vi "BESSY Put Test.vi"() -> ()   [LabVIEW 2011]
doc: "This Arbitrary Waveform Generator front panel is aimed primarily at the use of two reflectometer instruments at the ISIS Pulsed Neutron Facility at the Rutherford Appleton Laboratory. As such some variable items have been defaulted, and the code follows the standards of the Instrument Controls programming team."
uses:
  Labview Modules/Common/Utilities/Logo.llb/Logo.ctl
  Labview Modules/Common/Utilities/VI Control.llb/Control - Display State.ctl
  Labview Modules/Drivers/Tektronix AFG 3021B/AFG3021B - Controls.llb/AFG3021B - Trigger Button.ctl
  <userlib>/caLab/sub/caLabGet01.vi
  Labview Modules/Common/Utilities/Equal.llb/Equal - Error.vi
  <userlib>/caLab/sub/caLabPut21.vi
panel:
  out "Set Point Ind":dbl
  in  "Set Point":dbl
  in  "Exit":bool
  in  "Set":bool
  out "Message":string
  out "Activity":bool
  out "Error":errorcluster
  in  "Logo":T1
  # "Version 0.0.1"
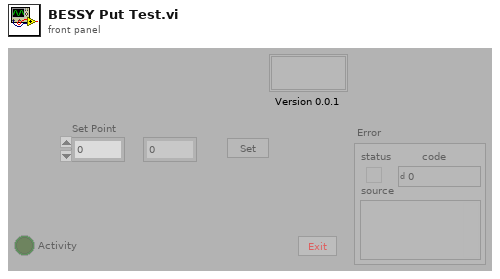
[diagram p1: front panel]
types:
  T1 = typedef "Logo.ctl" = u16
  T2 = typedef "Control - Display State.ctl" = enum16{"Enabled", "Disabled", "Disabled and Grayed"}
  T3 = typedef "AFG3021B - Trigger Button.ctl" = bool
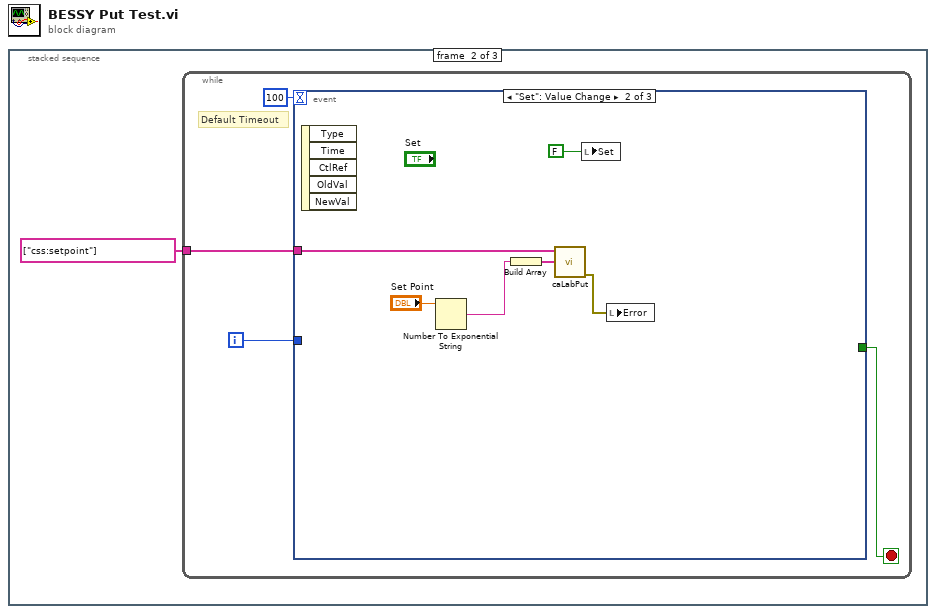
[diagram p0: block diagram]
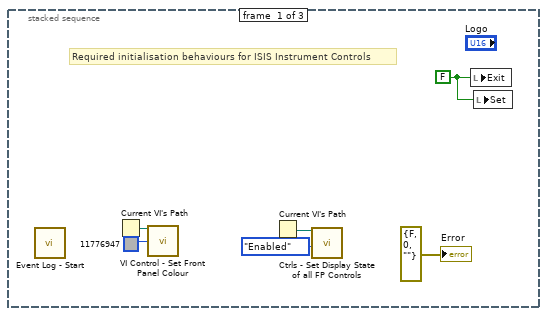
[diagram p2: hidden frame]
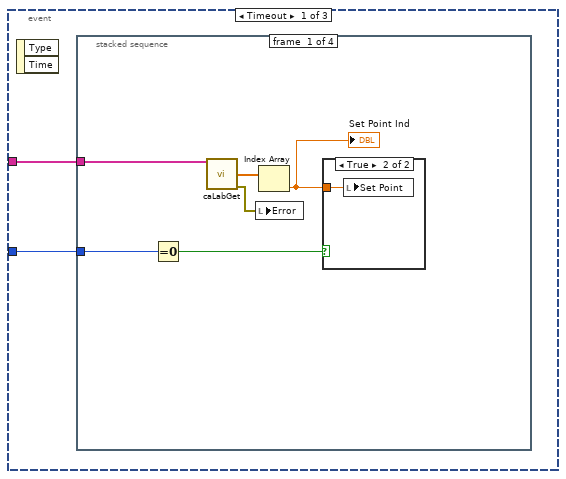
[diagram p3: hidden frame]
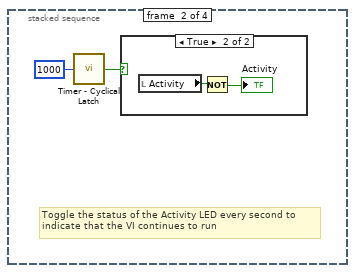
[diagram p5: hidden frame]
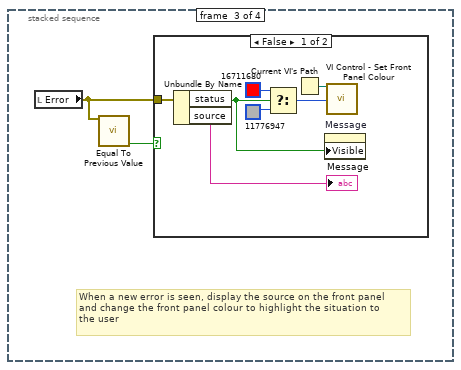
[diagram p7: hidden frame]
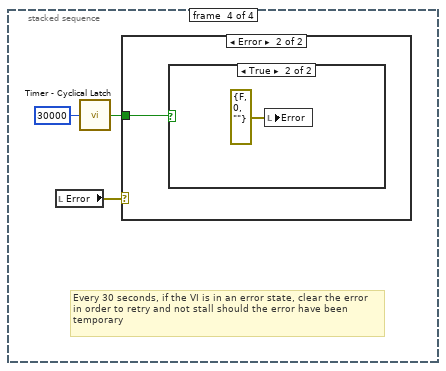
[diagram p9: hidden frame]
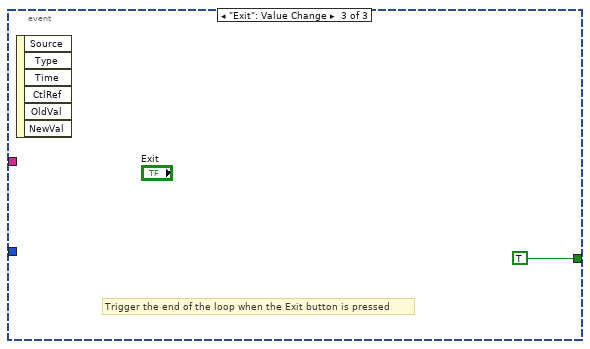
[diagram p12: hidden frame]
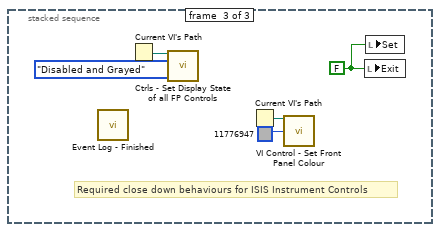
[diagram p13: hidden frame]
diagram:
  n1 = stacked-sequence {
    frame #0 {
      w1 = FALSE
      # "Required initialisation behaviours for ISIS Instrument Controls"
      n2 = call "Event Log - Start.vi"() -> ()  [unwired: 1 in]
      n3 = Current VI's Path() -> (path=w2:path)
      n4 = call "VI Control - Set Front Panel Colour.vi"("VI Path"=w2, "Front Panel Colour"=u32 11776947) -> ()  [unwired: 13 in, 1 out]
      n5 = Current VI's Path() -> (path=w6:path)
      n6 = call "Ctrls - Set Display State of all FP Controls.vi"("VI Path"=w6, "Display State"=Control_-_Display_State."Enabled") -> ()  [unwired: 18 in]
      n7 = local write "Exit"(w1) -> ()
      n8 = local write "Set"(w1) -> ()
      "Error" <- errorcluster {"status"=FALSE, "code"=0, "source"=""} ("Error")
    }
    frame #1 {
      n9 = while {
        tunnel: string[] ["css:setpoint"] ("PV name (array)") -> [w8]
        i -> [w9]
        stop <- w10 stop-if-true
        # "Default Timeout"
        n10 = event shown="[1] \"Set\": Value Change" {
          selector: _ -> [_ _ _]
          dyn-events: _ -> [_ _ _]
          timeout: 100 -> [_ _ _]
          tunnel: [_ _ TRUE] -> w10
          tunnel: w9 -> [w13 _ _]
          tunnel: w8 -> [w12 w43 _]
          event Timeout {
            n11 = event-data() -> ()  [unwired: 1 in, 2 out]
            n12 = stacked-sequence {
              tunnel: w13 -> [w19 _ _ _]
              tunnel: w12 -> [w14 _ _ _]
              frame #0 {
                n13 = Equal To 0?(x=w19) -> (x = 0?=w18:bool)
                n14 = call-poly <userlib>:"caLabGet.vi"("PV name (array)"=w14) -> ("1st value(number)"=w17:dbl[], "error out"=w15:errorcluster)  [unwired: 8 in, 5 out]
                n15 = local write "Error"(w15) -> ()
                n16 = Index Array(array=w17) -> (element=w16:dbl)  [unwired: 1 in]
                "Set Point Ind" <- w16
                n17 = case shown="True" w18 {
                  tunnel: w16 -> [_ w20]
                  frame False {
                  }
                  frame True {
                    n18 = local write "Set Point"(w20) -> ()
                  }
                }
              }
              frame #1 {
                # "Toggle the status of the Activity LED every second to\nindicate that the VI continues to run"
                n19 = call "Timer - Cyclical Latch.vi"("Timer (msec)"=u32 1000) -> ("Timer Trigger"=w21:bool)  [unwired: 14 in]
                n20 = case shown="True" w21 {
                  frame False {
                  }
                  frame True {
                    n21 = local read "Activity"() -> (w23:bool)
                    n22 = Not(x=w23) -> (.not. x?=→"Activity":bool)
                  }
                }
              }
              frame #2 {
                # "When a new error is seen, display the source on the front panel\nand change the front panel colour to highlight the situation to\nthe user"
                n23 = local read "Error"() -> (w26:errorcluster)
                n24 = call-poly "Equal To Previous Value.vi"("Value In"=w26) -> ("Equal to previous value"=w25:bool)  [unwired: 13 in, 1 out]
                n25 = case shown="False" w25 {
                  tunnel: w26 -> [w29 _]
                  frame False {
                    n26 = Unbundle By Name(w29) -> ("status"=w28:bool, "source"=→"Message":string)
                    n27 = Select(t=u32 16711680, s=w28, f=u32 11776947) -> (s? t:f=w30:u32)
                    n28 = Current VI's Path() -> (path=w33:path)
                    n29 = property on="Message" class="Str"("Visible"=w28) -> ()  [unwired: 2 in, 2 out]
                    n30 = call "VI Control - Set Front Panel Colour.vi"("VI Path"=w33, "Front Panel Colour"=w30) -> ()  [unwired: 13 in, 1 out]
                  }
                  frame True {
                  }
                }
              }
              frame #3 {
                # "Every 30 seconds, if the VI is in an error state, clear the error\nin order to retry and not stall should the error have been \ntemporary"
                n31 = local read "Error"() -> (w35:errorcluster)
                n32 = call "Timer - Cyclical Latch.vi"("Timer (msec)"=u32 30000) -> ("Timer Trigger"=w34:bool)  [unwired: 14 in]
                n33 = case shown="Error" w35 {
                  tunnel: w34 -> [_ w37]
                  frame No Error {
                  }
                  frame Error {
                    n34 = case shown="True" w37 {
                      frame False {
                      }
                      frame True {
                        n35 = local write "Error"(errorcluster {"status"=FALSE, "code"=0, "source"=""} ("Error")) -> ()
                      }
                    }
                  }
                }
              }
            }
          }
          event "Set": Value Change {
            n36 = event-data() -> ()  [unwired: 1 in, 5 out]
            n37 = Number To Exponential String(number="Set Point") -> (E-format string=w39:string)  [unwired: 3 in]
            n38 = Build Array(w39) -> (w41:string[])
            n39 = call-poly <userlib>:"caLabPut.vi"("values"=w41, "PV name(s)"=w43) -> ("error out"=w42:errorcluster)  [unwired: 6 in, 3 out]
            n40 = local write "Set"(T3 FALSE ("Trigger")) -> ()
            n41 = local write "Error"(w42) -> ()
          }
          event "Exit": Value Change {
            # "Trigger the end of the loop when the Exit button is pressed"
            n42 = event-data() -> ()  [unwired: 1 in, 6 out]
          }
        }
      }
    }
    frame #2 {
      w46 = FALSE
      # "Required close down behaviours for ISIS Instrument Controls"
      n43 = call "Event Log - Finished.vi"() -> ()  [unwired: 1 in]
      n44 = Current VI's Path() -> (path=w49:path)
      n45 = call "Ctrls - Set Display State of all FP Controls.vi"("VI Path"=w49, "Display State"=Control_-_Display_State."Disabled and Grayed") -> ()  [unwired: 18 in]
      n46 = Current VI's Path() -> (path=w48:path)
      n47 = call "VI Control - Set Front Panel Colour.vi"("VI Path"=w48, "Front Panel Colour"=u32 11776947) -> ()  [unwired: 13 in, 1 out]
      n48 = local write "Exit"(w46) -> ()
      n49 = local write "Set"(w46) -> ()
    }
  }
